vi "VisitSites.vi"(0 "Microsites":T3(array[cluster]), 4 "Path":path, 7 "UiDefinition":T2, 13 "CurrentPositionIndex":i32) -> ()   [LabVIEW 2020]
uses:
  UIReferences.ctl
  D:/LabviewDXFViewer/LabviewDXFViewer/bin/Release/LabviewDXFViewer.exe
  LabviewDXFViewer/bin/Release/LabviewDXFViewer.exe
  Control 2.ctl
  <vilib>/Utility/file.llb/Write Delimited Spreadsheet (string).vi
panel:
  out "error out 17":errorcluster
  out "error out 16":errorcluster
  out "error out 15":errorcluster
  out "error out 14":errorcluster
  out "error out 13":errorcluster
  out "error out 12":errorcluster
  out "error out 11":errorcluster
  out "error out 10":errorcluster
  out "error out 9":errorcluster
  out "error out 8":errorcluster
  out "error out 7":errorcluster
  out "error out 6":errorcluster
  out "error out 5":errorcluster
  out "error out 4":errorcluster
  out "IV Curves":T1
  out "error out 3":errorcluster
  out "error out 2":errorcluster
  out "error out":errorcluster
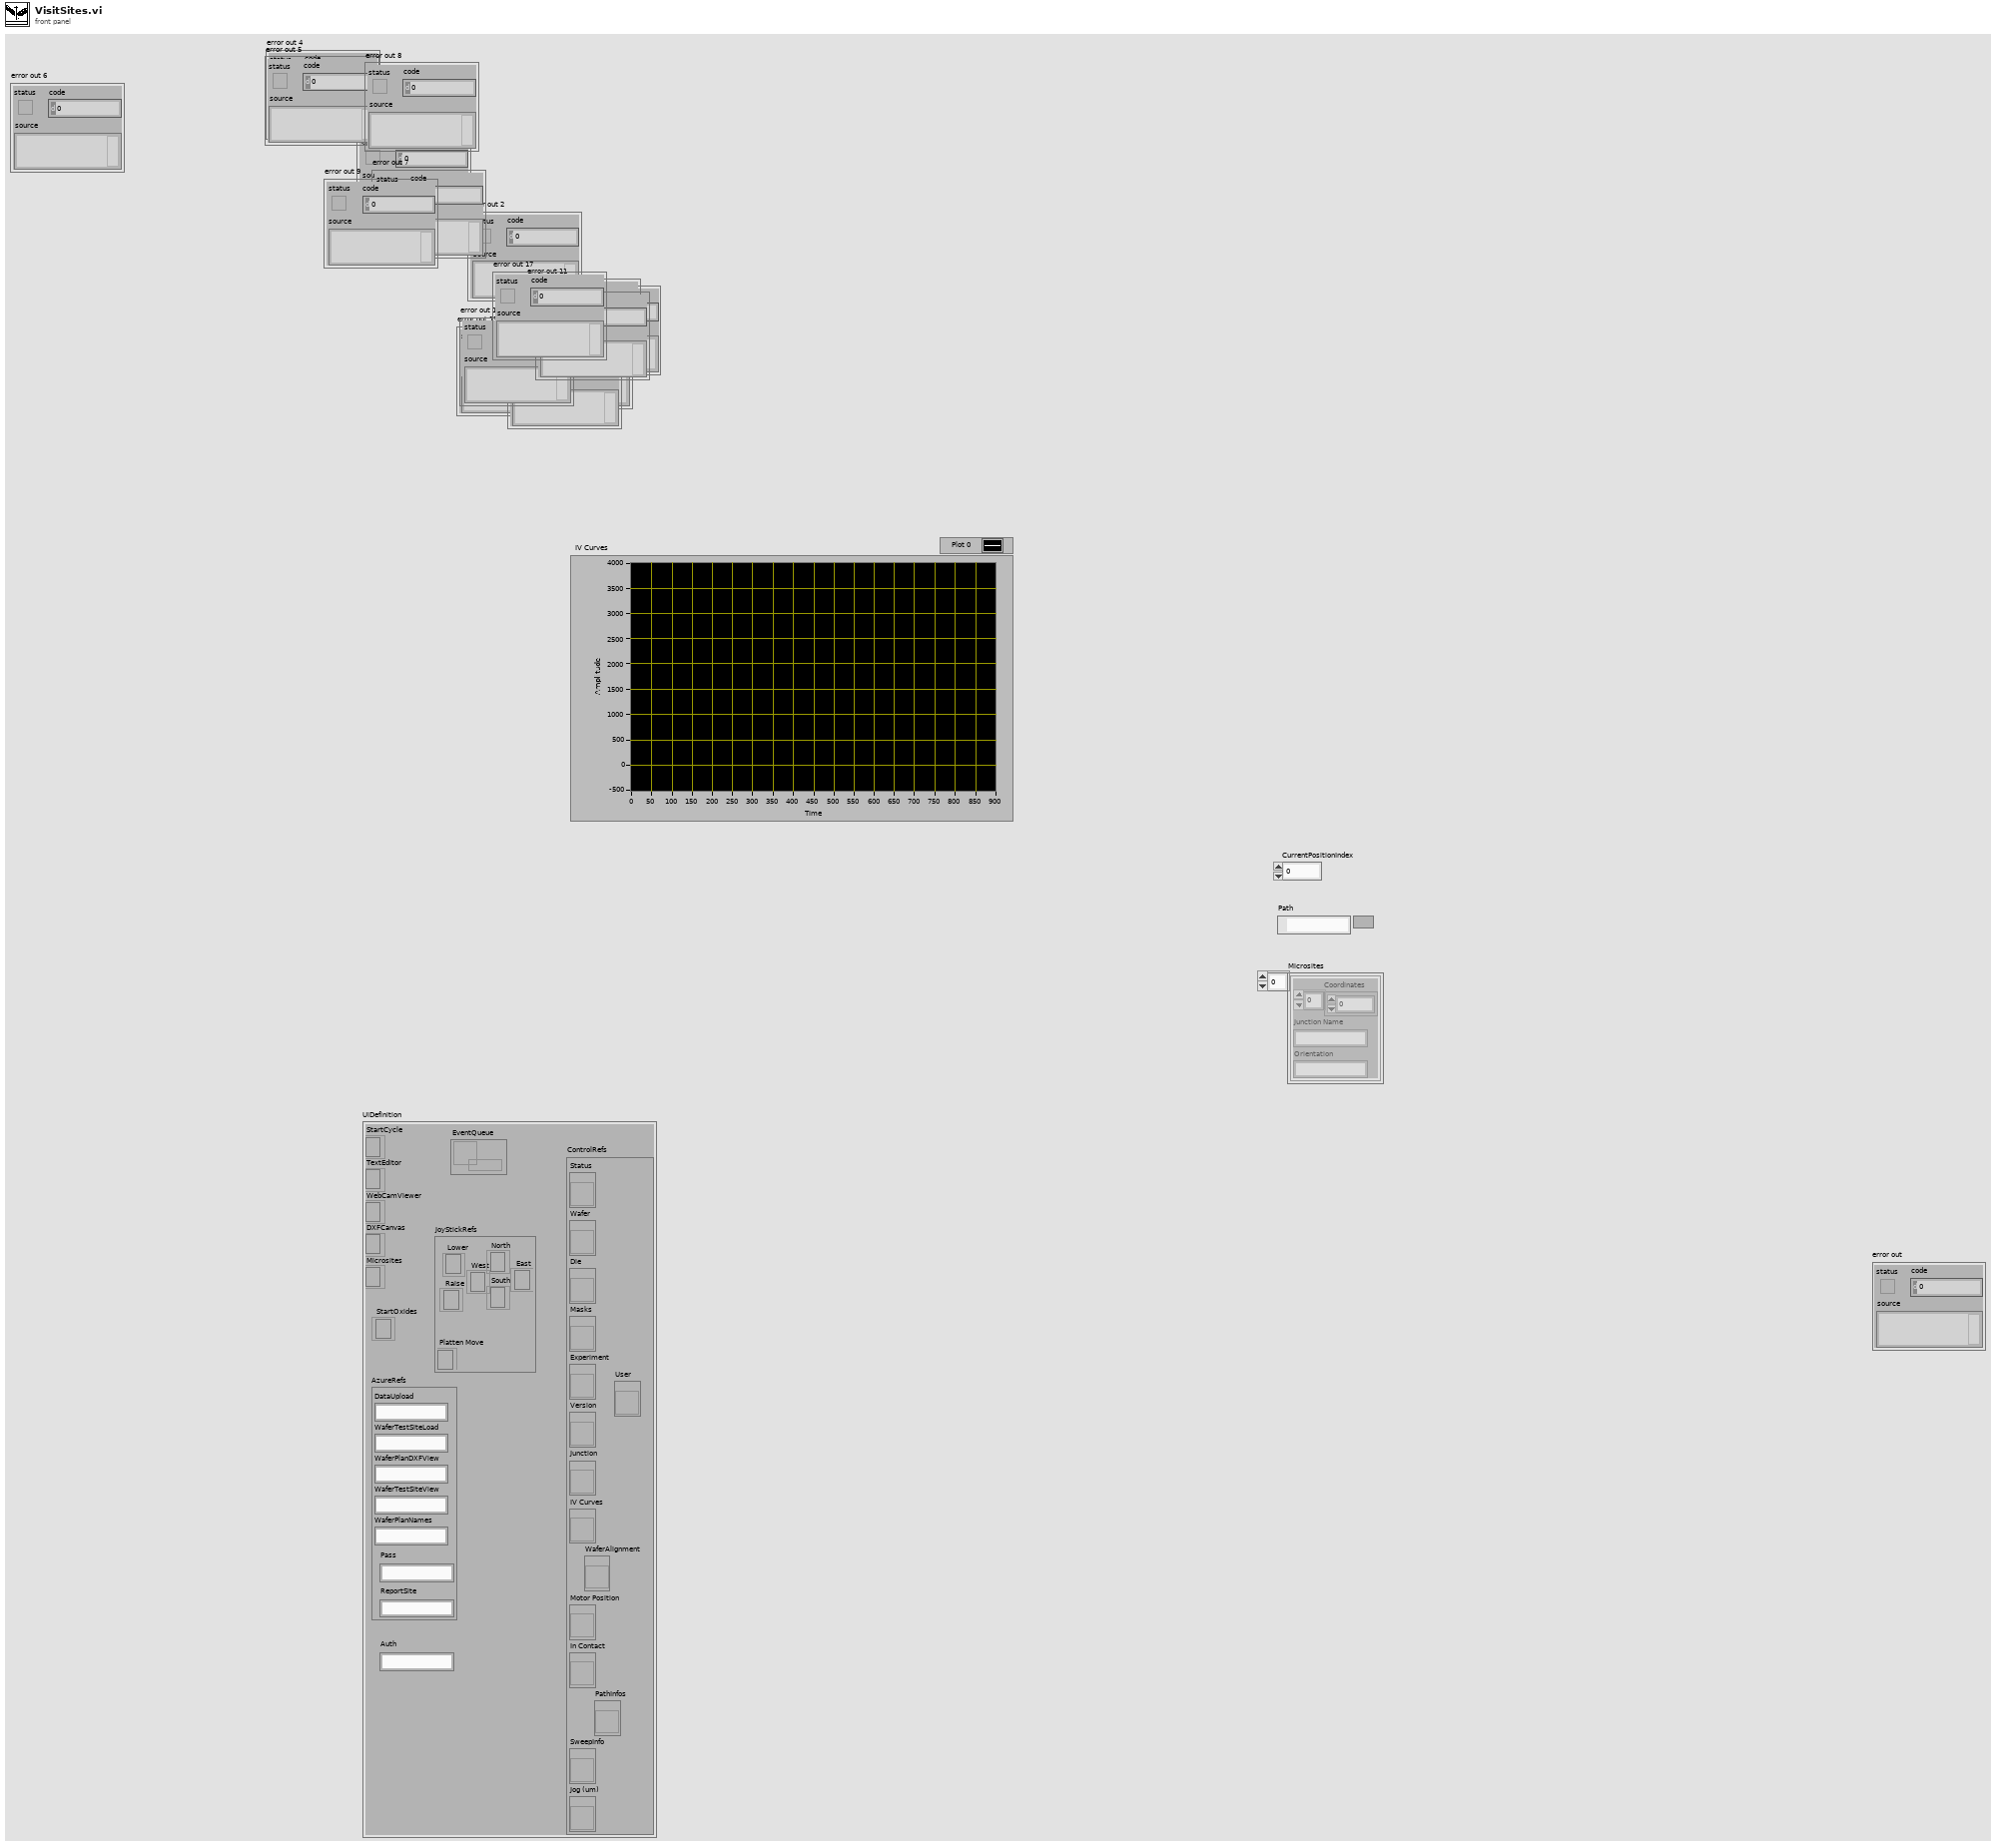
[diagram p1: front panel]
types:
  T1 = typedef "Control 2.ctl" = cluster{"Y":dbl[], "Current (A)":dbl[]}
  T2 = typedef "UIReferences.ctl" = cluster{"StartCycle":refnum<k24>, "TextEditor":refnum<k24>, "WebCamViewer":refnum<k24>, "DXFCanvas":refnum<k24>, "Microsites":refnum<k24>, "JoyStickRefs":cluster{"North":refnum<k24>, "Lower":refnum<k24>, "Raise":refnum<k24>, "Platten Move":refnum<k24>, "West":refnum<k24>, "East":refnum<k24>, "South":refnum<k24>}, "AzureRefs":cluster{"DataUpload":string, "WaferTestSiteLoad":string, "WaferPlanDXFView":string, "WaferTestSiteView":string, "WaferPlanNames":string, "Pass":string, "ReportSite":string}, "ControlRefs":cluster{"Status":refnum<vi>, "Wafer":refnum<vi>, "Die":refnum<vi>, "Masks":refnum<vi>, "Experiment":refnum<vi>, "Version":refnum<vi>, "Junction":refnum<vi>, "IV Curves":refnum<vi>, "Motor Position":refnum<vi>, "In Contact":refnum<vi>, "SweepInfo":refnum<vi>, "Jog (um)":refnum<vi>, "PathInfos":refnum<vi>, "User":refnum<vi>, "WaferAlignment":refnum<vi>}, "EventQueue":refnum<queue>, "StartOxides":refnum<k24>, "Auth":string}
  T3 = cluster{"Coordinates":dbl[], "Junction Name":string, "Orientation":string}[]
  T4 = cluster{"Coordinates":dbl[], "Junction Name":string, "Orientation":string}
  T5 = typedef "WaferAlignmentType.ctl" = cluster{"Wafer Units to microns":dbl, "Rotation Misalign":dbl[], "Scale Misalign":dbl, "Steps Per micron":dbl, "Position 1":i32[], "Position 2":i32[], "Lift Distance":i32, "Position 3":i32[], "Jog Height":i32}
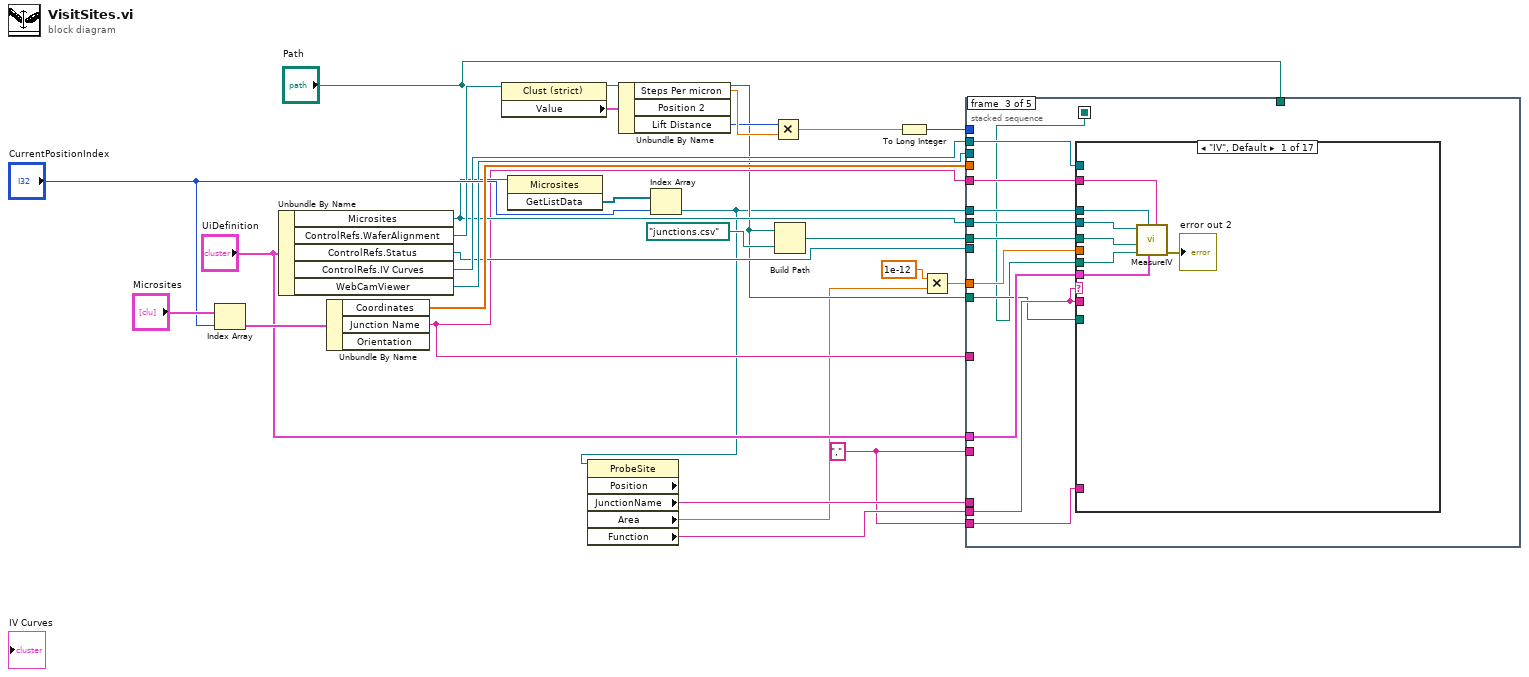
[diagram p0: block diagram]
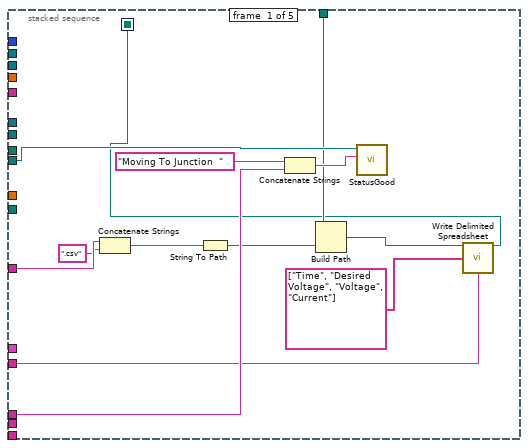
[diagram p2: hidden frame]
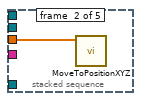
[diagram p3: hidden frame]
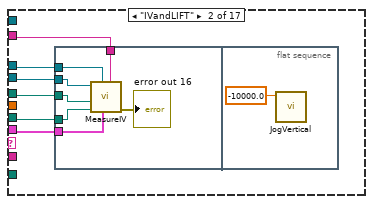
[diagram p4: hidden frame]
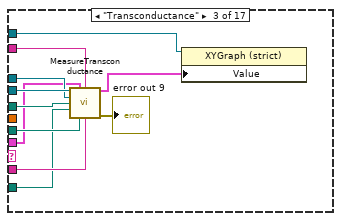
[diagram p5: hidden frame]
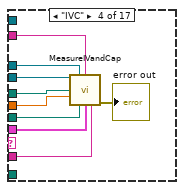
[diagram p6: hidden frame]
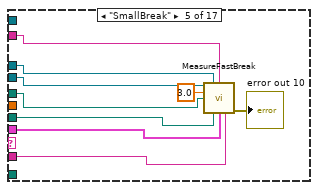
[diagram p7: hidden frame]
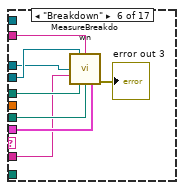
[diagram p8: hidden frame]
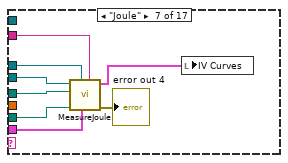
[diagram p9: hidden frame]
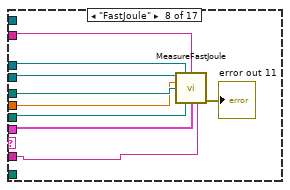
[diagram p10: hidden frame]
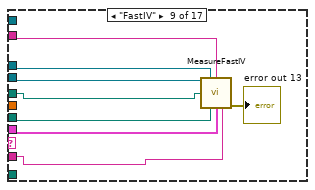
[diagram p11: hidden frame]
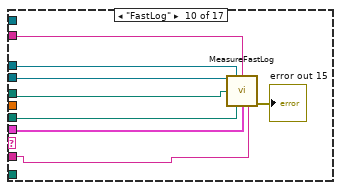
[diagram p12: hidden frame]
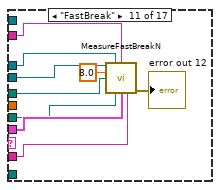
[diagram p13: hidden frame]
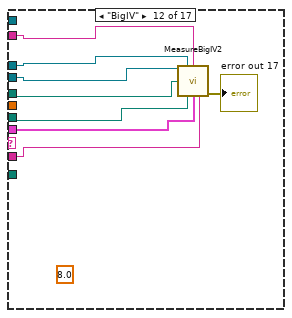
[diagram p14: hidden frame]
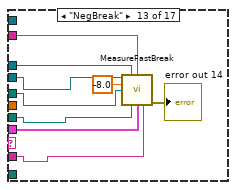
[diagram p15: hidden frame]
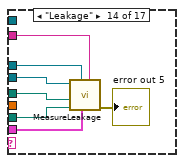
[diagram p16: hidden frame]
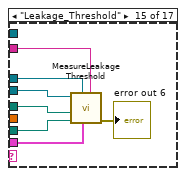
[diagram p17: hidden frame]
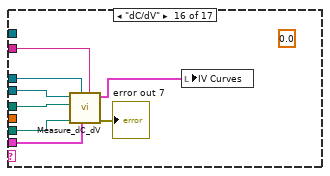
[diagram p18: hidden frame]
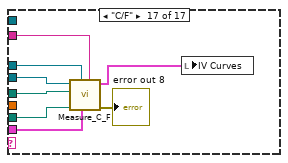
[diagram p19: hidden frame]
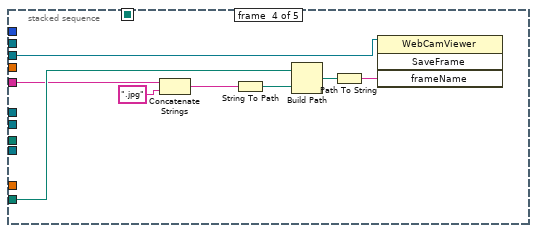
[diagram p20: hidden frame]
diagram:
  w5 = "," ("delimiter (\\t)")
  n1 = Index Array(array="Microsites", index="CurrentPositionIndex") -> (element=w22:T4)
  n2 = Unbundle By Name("UiDefinition") -> ("Microsites"=w8:refnum<k24>, "ControlRefs.WaferAlignment"=w19:refnum<vi>, "ControlRefs.Status"=w6:refnum<vi>, "ControlRefs.IV Curves"=w14:refnum<vi>, "WebCamViewer"=w12:refnum<k24>)
  n3 = Unbundle By Name(w22) -> ("Coordinates"=w25:dbl[], "Junction Name"=w4:string)  [unwired: 1 out]
  n4 = property class="Clust (strict)"(reference=w19) -> ("Value"=w18:T5)  [unwired: 1 in, 2 out]
  n5 = invoke class="Microsites" method="GetListData"(reference=w8) -> ("GetListData"=w20:refnum<k24>[])  [unwired: 2 in, 2 out]
  n6 = Unbundle By Name(w18) -> ("Steps Per micron"=w16:dbl, "Lift Distance"=w15:i32)  [unwired: 1 out]
  n7 = Index Array(array=w20, index="CurrentPositionIndex") -> (element=w1:refnum<k24>)
  n8 = property class="ProbeSite" props=["Position", "JunctionName", "Area", "Function"](reference=w1) -> ("JunctionName"=w7:string, "Area"=w2:dbl, "Function"=w9:string)  [unwired: 1 in, 3 out]
  n9 = Multiply(x=w15, y=w16) -> (x*y=w17:dbl)
  n10 = Build Path(base path="Path", name or relative path=path "junctions.csv") -> (appended path=w26:path)
  n11 = To Long Integer(number=w17) -> (32bit integer=w27:i32)
  n12 = Multiply(x=1e-12, y=w2) -> (x*y=w11:dbl)
  n13 = stacked-sequence {
    seq-local: [w28 _ _ _ _] -> [_ _ w42 _ _]
    tunnel: w27 -> [_ _ _ _ w209]
    tunnel: w26 -> [_ _ w52 _ _]
    tunnel: w25 -> [_ w41 _ _ _]
    tunnel: w4 -> [_ _ w51 w202 _]
    tunnel: w14 -> [_ _ w44 _ _]
    tunnel: "UiDefinition" -> [_ _ w49 _ _]
    tunnel: w5 -> [_ _ w50 _ _]
    tunnel: w12 -> [_ _ _ w207 _]
    tunnel: "Path" -> [_ _ w43 w206 _]
    tunnel: w11 -> [_ _ w48 _ _]
    tunnel: w9 -> [_ _ w45 _ _]
    tunnel: w8 -> [_ _ w47 _ _]
    tunnel: w1 -> [_ _ w46 _ _]
    tunnel: w7 -> [w38 _ _ _ _]
    tunnel: w6 -> [w37 _ _ _ _]
    tunnel: w5 -> [w32 _ _ _ _]
    tunnel: w4 -> [w31 _ _ _ _]
    tunnel: "Path" -> [w29 _ _ _ _]
    frame #0 {
      n14 = Concatenate Strings(w31, ".csv" ("string")) -> (w34:string)
      n15 = String To Path(string=w34) -> (path=w35:path)
      n16 = Concatenate Strings("Moving To Junction  " ("Text.Text"), w38) -> (w40:string)
      n17 = Build Path(base path=w29, name or relative path=w35) -> (appended path=w36:path)
      n18 = call "StatusGood.vi"("Text.Text"=w40, "String in"=w37) -> ()  [unwired: 10 in]
      n19 = call-poly <vilib>:"Write Delimited Spreadsheet.vi"("file path (dialog if empty)"=w36, "1D data"=string[] ["Time", "Desired Voltage", "Voltage", "Current"], "delimiter (\\t)"=w32) -> ("new file path (Not A Path if cancelled)"=w28:path)  [unwired: 11 in, 1 out]
    }
    frame #1 {
      n20 = call "MoveToPositionXYZ.vi"("Array"=w41) -> ()  [unwired: 11 in]
    }
    frame #2 {
      n21 = case shown="\"IV\", Default" w45 {
        tunnel: w52 -> [w57 w62 w80 w93 w94 w110 w113 w121 w131 w139 w144 w156 w162 w173 w179 w188 w196]
        tunnel: w51 -> [w56 w65 w74 w92 w101 w104 w114 w126 w134 w142 w151 w155 w167 w172 w180 w187 w195]
        tunnel: w42 -> [w58 w61 w81 w91 w96 w109 w115 w120 w130 w138 w146 w157 w161 w171 w178 w186 w193]
        tunnel: w50 -> [_ _ _ _ _ _ _ _ _ _ _ _ _ _ _ _ _]
        tunnel: w49 -> [w55 w60 w78 w90 w97 w106 w112 w122 w129 w137 w147 w158 w164 w170 w177 w185 w194]
        tunnel: w48 -> [_ _ _ w89 _ _ _ w119 _ _ _ _ _ _ _ _ _]
        tunnel: w47 -> [w54 w63 w83 w88 w99 w108 w117 w124 w132 w140 w149 w153 w163 w174 w181 w189 w197]
        tunnel: w46 -> [w53 w64 w82 w87 w100 w107 w116 w125 w133 w141 w150 w154 w166 w175 w182 w190 w198]
        tunnel: w45 -> [_ _ w79 w86 w98 w105 _ w123 w128 w136 w148 w159 w165 _ _ _ _]
        tunnel: w44 -> [_ _ w77 _ _ _ _ _ _ _ _ _ _ _ _ _ _]
        tunnel: w43 -> [_ _ w75 _ _ _ _ _ _ _ _ _ _ _ _ _ _]
        frame "IV", Default {
          n22 = call "MeasureIV.vi"("Junction Name"=w56, "UiDefinition"=w55, ".NET Refnum"=w53, "new file path (Not A Path if cancelled)"=w58, "appended path"=w57, ".NET Refnum in"=w54) -> ("error out"=→"error out 2":errorcluster)  [unwired: 5 in]
        }
        frame "IVandLIFT" {
          n23 = flat-sequence {
            tunnel: w65 -> [w71]
            tunnel: w64 -> [w70]
            tunnel: w63 -> [w69]
            tunnel: w62 -> [w68]
            tunnel: w61 -> [w67]
            tunnel: w60 -> [w66]
            frame #0 {
              n24 = call "MeasureIV.vi"("Junction Name"=w71, "UiDefinition"=w66, ".NET Refnum"=w70, "new file path (Not A Path if cancelled)"=w67, "appended path"=w68, ".NET Refnum in"=w69) -> ("error out"=→"error out 16":errorcluster)  [unwired: 5 in]
            }
            frame #1 {
              n25 = call "JogVertical.vi"("Numeric"=-10000.0) -> ()  [unwired: 11 in]
            }
          }
        }
        frame "Transconductance" {
          n26 = call "MeasureTransconductance.vi"(".NET Refnum in"=w83, "UiDefinition"=w78, "Junction Name"=w74, ".NET Refnum"=w82, "appended path"=w80, "Path"=w75, "new file path (Not A Path if cancelled)"=w81, "Function"=w79) -> ("Cluster"=w76:cluster{dbl[], dbl[]}, "error out"=→"error out 9":errorcluster)  [unwired: 6 in]
          n27 = property class="XYGraph (strict)"(reference=w77, "Value"=w76) -> ()  [unwired: 1 in, 2 out]
        }
        frame "IVC" {
          n28 = call "MeasureIVandCap.vi"(".NET Refnum in"=w88, ".NET Refnum"=w87, "Junction Name"=w92, "appended path"=w93, "Numeric"=w89, "new file path (Not A Path if cancelled)"=w91, "UiDefinition"=w90, "Function"=w86) -> ("error out"=→"error out":errorcluster)  [unwired: 7 in]
        }
        frame "SmallBreak" {
          n29 = call "MeasureFastBreak.vi"(".NET Refnum in"=w99, ".NET Refnum"=w100, "Junction Name"=w101, "Maxiumum Voltage"=3.0, "appended path"=w94, "new file path (Not A Path if cancelled)"=w96, "UiDefinition"=w97, "Function"=w98) -> ("error out"=→"error out 10":errorcluster)  [unwired: 7 in]
        }
        frame "Breakdown" {
          n30 = call "MeasureBreakdown.vi"("Microsites"=w108, "Junction Name"=w104, ".NET Refnum"=w107, "Function"=w105, "appended path"=w110, "new file path (Not A Path if cancelled)"=w109, "UiDefinition"=w106) -> ("error out"=→"error out 3":errorcluster)  [unwired: 8 in]
        }
        frame "Joule" {
          n31 = call "MeasureJoule.vi"("Junction Name"=w114, "UiDefinition"=w112, ".NET Refnum"=w116, "new file path (Not A Path if cancelled)"=w115, "appended path"=w113, ".NET Refnum in"=w117) -> ("error out"=→"error out 4":errorcluster, "Cluster"=w111:cluster{dbl[], dbl[]})  [unwired: 4 in]
          n32 = local write "IV Curves"(w111) -> ()
        }
        frame "FastJoule" {
          n33 = call "MeasureFastJoule.vi"(".NET Refnum in"=w124, ".NET Refnum"=w125, "Junction Name"=w126, "Maxiumum Voltage"=w119, "appended path"=w121, "new file path (Not A Path if cancelled)"=w120, "UiDefinition"=w122, "Function"=w123) -> ("error out"=→"error out 11":errorcluster)  [unwired: 7 in]
        }
        frame "FastIV" {
          n34 = call "MeasureFastIV.vi"(".NET Refnum in"=w132, ".NET Refnum"=w133, "Junction Name"=w134, "appended path"=w131, "new file path (Not A Path if cancelled)"=w130, "UiDefinition"=w129, "Function"=w128) -> ("error out"=→"error out 13":errorcluster)  [unwired: 8 in]
        }
        frame "FastLog" {
          n35 = call "MeasureFastLog.vi"(".NET Refnum in"=w140, ".NET Refnum"=w141, "Junction Name"=w142, "appended path"=w139, "new file path (Not A Path if cancelled)"=w138, "UiDefinition"=w137, "Function"=w136) -> ("error out"=→"error out 15":errorcluster)  [unwired: 8 in]
        }
        frame "FastBreak" {
          n36 = call "MeasureFastBreakN.vi"(".NET Refnum in"=w149, ".NET Refnum"=w150, "Junction Name"=w151, "MaxVoltage"=8.0 ("Maxiumum Voltage"), "appended path"=w144, "new file path (Not A Path if cancelled)"=w146, "UiDefinition"=w147, "Function"=w148) -> ("error out"=→"error out 12":errorcluster)  [unwired: 7 in]
        }
        frame "BigIV" {
          (unwired) 8.0 ("Maxiumum Voltage")
          n37 = call "MeasureBigIV2.vi"(".NET Refnum in"=w153, ".NET Refnum"=w154, "Junction Name"=w155, "appended path"=w156, "new file path (Not A Path if cancelled)"=w157, "UiDefinition"=w158, "Function"=w159) -> ("error out"=→"error out 17":errorcluster)  [unwired: 8 in]
        }
        frame "NegBreak" {
          n38 = call "MeasureFastBreak.vi"(".NET Refnum in"=w163, ".NET Refnum"=w166, "Junction Name"=w167, "Maxiumum Voltage"=-8.0, "appended path"=w162, "new file path (Not A Path if cancelled)"=w161, "UiDefinition"=w164, "Function"=w165) -> ("error out"=→"error out 14":errorcluster)  [unwired: 7 in]
        }
        frame "Leakage" {
          n39 = call "MeasureLeakage.vi"("Junction Name"=w172, "UiDefinition"=w170, ".NET Refnum"=w175, "new file path (Not A Path if cancelled)"=w171, "appended path"=w173, ".NET Refnum in"=w174) -> ("error out"=→"error out 5":errorcluster)  [unwired: 5 in]
        }
        frame "Leakage_Threshold" {
          n40 = call "MeasureLeakageThreshold.vi"("Junction Name"=w180, "UiDefinition"=w177, ".NET Refnum"=w182, "new file path (Not A Path if cancelled)"=w178, "appended path"=w179, ".NET Refnum in"=w181) -> ("error out"=→"error out 6":errorcluster)  [unwired: 5 in]
        }
        frame "dC/dV" {
          (unwired) 0.0 ("Vpp")
          n41 = call "Measure_dC_dV.vi"("Junction Name"=w187, "UiDefinition"=w185, ".NET Refnum"=w190, "new file path (Not A Path if cancelled)"=w186, "appended path"=w188, ".NET Refnum in"=w189) -> ("error out"=→"error out 7":errorcluster, "Cluster"=w184:cluster{dbl[], dbl[]})  [unwired: 4 in]
          n42 = local write "IV Curves"(w184) -> ()
        }
        frame "C/F" {
          n43 = call "Measure_C_F.vi"("Junction Name"=w195, "UiDefinition"=w194, ".NET Refnum"=w198, "new file path (Not A Path if cancelled)"=w193, "appended path"=w196, ".NET Refnum in"=w197) -> ("error out"=→"error out 8":errorcluster, "Cluster"=w192:cluster{dbl[], dbl[]})  [unwired: 4 in]
          n44 = local write "IV Curves"(w192) -> ()
        }
      }
    }
    frame #3 {
      n45 = Concatenate Strings(w202, ".jpg" ("string")) -> (w205:string)
      n46 = String To Path(string=w205) -> (path=w203:path)
      n47 = Build Path(base path=w206, name or relative path=w203) -> (appended path=w201:path)
      n48 = Path To String(path=w201) -> (string=w200:string)
      n49 = invoke class="WebCamViewer" method="SaveFrame"(reference=w207, "frameName"=w200) -> ()  [unwired: 2 in, 4 out]
    }
    frame #4 {
      # "Move Up"
      n50 = Negate(x=w209) -> (-x=w208:i32)
      n51 = call "JogVertical.vi"("Numeric"=w208) -> ()  [unwired: 11 in]
    }
  }
